vi "test_g4_type.vi"() -> ()   [LabVIEW 2017, in "labview-standard-library.lvlib" / "automode-scripting.lvlib"]
uses:
  automode-scripting.lvlib
  type-defs/execution_stop_type.ctl
panel:
  out "Array":T1[](array[typedef])
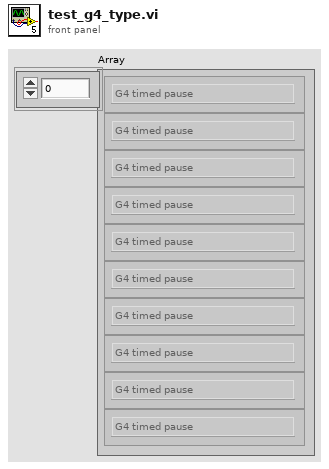
[diagram p1: front panel]
types:
  T1 = typedef "labview-standard-library.lvlib/automode-scripting.lvlib/execution_stop_type.ctl" = enum16{"G4 timed pause", "G4 previous line pause", "G4 tool pause", "Invalid"}
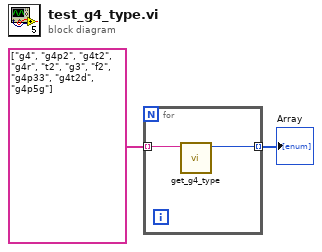
[diagram p0: block diagram]
diagram:
  n1 = for {
    tunnel: [w4] -> w1 mode=indexing
    tunnel: string[] ["g4", "g4p2", "g4t2", "g4r", "t2", "g3", "f2", "g4p33", "g4t2d", "g4p5g"] -> [w3] mode=indexing
    n2 = call "get_g4_type.vi"("Line in"=w3) -> ("G4 type"=w4:T1)  [unwired: 9 in, 1 out]
  }
  "Array" <- w1
